vi "Conver Encoder distance to ft.vi"(6 "RevMotor/RevWheel":dbl=6.67 format="%#_13g", 7 "New CMD":bool, 8 "Wheel Diameter (in)":dbl=4.0 format="%#_13g", 9 "CPR (Ct/Rev Mot)":dbl=2048.0, 10 "Drive Position Values":i32[](array[numeric]), 11 "Drive Position Offsets":i32[](array[numeric])) -> (2 "Calculated Ft Out":dbl, 3 "Drive Position Offsets Out":i32[](array[numeric]))   [LabVIEW 2020, in "SwerveDrive_ACT.lvlib"]
uses:
  SwerveDrive_ACT.lvlib
panel:
  out "x-y":i32[](array[numeric])
  out "avg pos":i32
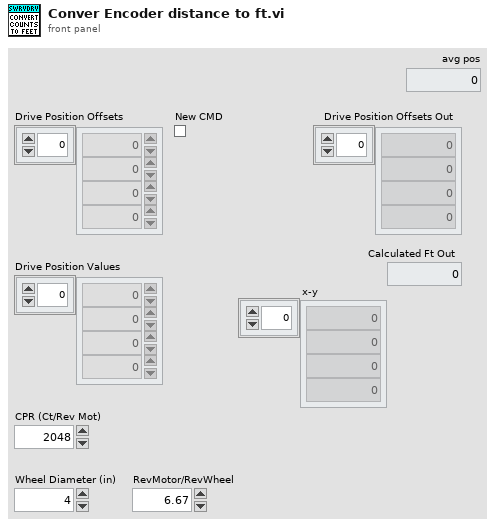
[diagram p1: front panel]
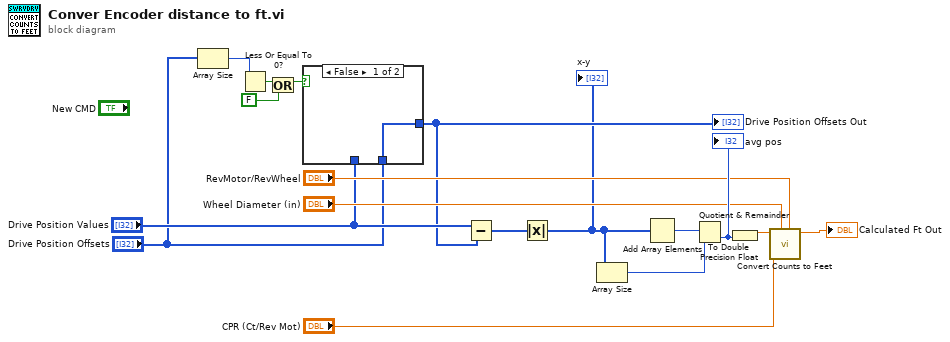
[diagram p0: block diagram]
diagram:
  n1 = Array Size(array="Drive Position Offsets") -> (size(s)=w7:i32)
  n2 = Less Or Equal To 0?(x=w7) -> (x <= 0?=w6:bool)
  n3 = Or(x=w6, y=FALSE) -> (x .or. y?=w5:bool)
  n4 = case shown="False" w5 {
    tunnel: "Drive Position Values" -> [_ w19]
    tunnel: "Drive Position Offsets" -> [w18 _]
    tunnel: [w18 w19] -> w2
    frame False {
    }
    frame True {
      # "Reset Distance"
    }
  }
  "Drive Position Offsets Out" <- w2
  n5 = Subtract(x="Drive Position Values", y=w2) -> (x-y=w3:i32[])
  n6 = Absolute Value(x=w3) -> (abs(x)=w1:i32[])
  "x-y" <- w1
  n7 = Array Size(array=w1) -> (size(s)=w16:i32)
  n8 = Add Array Elements(numeric array=w1) -> (sum=w17:i32)
  n9 = Quotient & Remainder(x=w17, y=w16) -> (floor(x/y)=w15:i32)  [unwired: 1 out]
  "avg pos" <- w15
  n10 = To Double Precision Float(number=w15) -> (double precision float=w10:dbl)
  n11 = call "Convert Counts to Feet.vi"("RevMotor/RevWheel"="RevMotor/RevWheel", "Wheel Diameter (in)"="Wheel Diameter (in)", "CPR (Ct/Rev mot)"="CPR (Ct/Rev Mot)", "Counts"=w10) -> ("Ft"=→"Calculated Ft Out":dbl)  [unwired: 7 in]
